vi "EsingleGenerator.vi"(10 "Numeric in":i32, 11 "Boolean":bool) -> (3 "Numeric out":dbl)   [LabVIEW 2024]
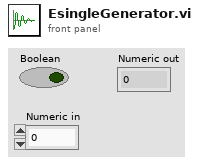
[diagram p1: front panel]
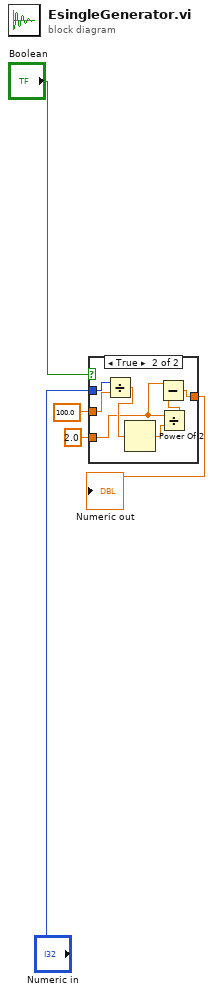
[diagram p0: block diagram]
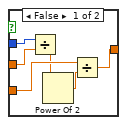
[diagram p2: hidden frame]
diagram:
  n1 = case shown="True" "Boolean" {
    tunnel: [w11 w18] -> w5
    tunnel: 2.0 -> [w10 w12]
    tunnel: 100.0 -> [w9 w16]
    tunnel: "Numeric in" -> [w8 w15]
    frame False {
      n2 = Divide(x=w8, y=w9) -> (x/y=w7:dbl)
      n3 = Power Of 2(x=w7) -> (2^x=w6:dbl)
      n4 = Divide(x=w10, y=w6) -> (x/y=w11:dbl)
    }
    frame True {
      n5 = Divide(x=w15, y=w16) -> (x/y=w14:dbl)
      n6 = Power Of 2(x=w14) -> (2^x=w13:dbl)
      n7 = Divide(x=w12, y=w13) -> (x/y=w17:dbl)
      n8 = Subtract(x=w12, y=w17) -> (x-y=w18:dbl)
    }
  }
  "Numeric out" <- w5
